vi "transform_axis_positions.vi"(6 "Current status":T1={"Axis names"=["X", "Y", "Z", "Rx", "Ry", "Rz"], "Axis positions"=[], "Pose"=[], "Timestamp"=0, "Ready"=FALSE, "Stopped"=FALSE} {"Pose" format="%#.4f"; "Axis positions" format="%#.4f"}, 8 "error in":errorcluster, 11 "Command":T2) -> (0 "error out":errorcluster, 1 "Absolute":bool, 2 "Axis positions":dbl[](array[numeric]), 3 "Axis enable":bool[](array[boolean]), 4 "Final status":T1={"Axis names"=["X", "Y", "Z", "Rx", "Ry", "Rz"], "Axis positions"=[], "Pose"=[], "Timestamp"=0, "Ready"=FALSE, "Stopped"=FALSE} {"Pose" format="%#.4f"; "Axis positions" format="%#.4f"})   [LabVIEW 2024]
uses:
  motion_command.ctl
  motion_status.ctl
  <vilib>/Analysis/baseanly.llb/Real A x B.vi
  <vilib>/Analysis/NI_AALBase.lvlib
panel:
  # "Do inverse kinematics, etc., to generate the inputs to the low-level motion drivers."
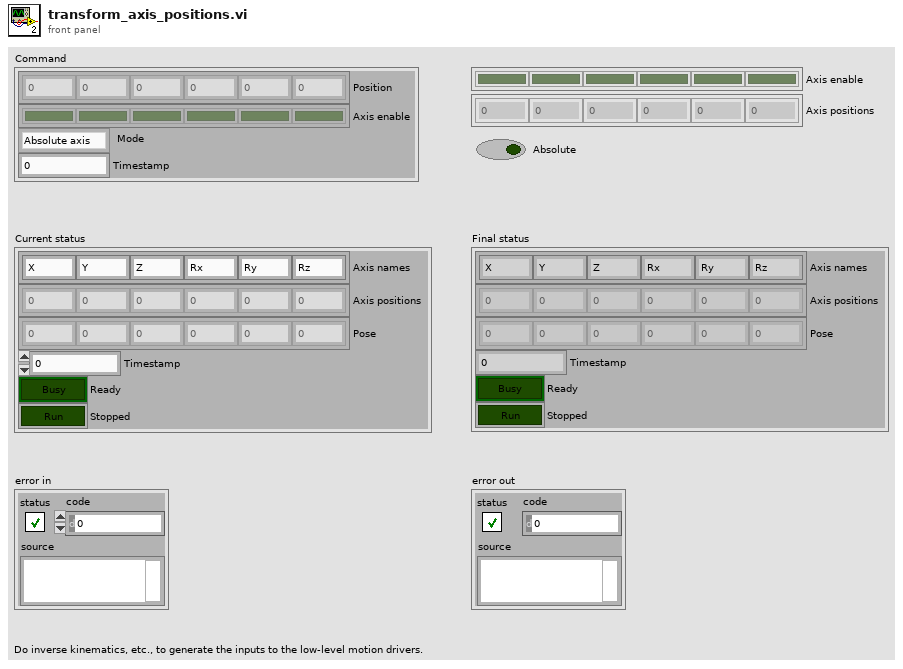
[diagram p1: front panel]
types:
  T1 = typedef "motion_status.ctl" = cluster{"Axis names":string[], "Axis positions":dbl[], "Pose":dbl[], "Timestamp":u32, "Ready":bool, "Stopped":bool}
  T2 = typedef "motion_command.ctl" = cluster{"Position":dbl[], "Axis enable":bool[], "Mode":enum16{"Absolute axis", "Relative axis", "Pose"}, "Timestamp":u32}
  T3 = typedef "NI_Matrix.lvlib/RealMatrix.ctl" = dbl[][]
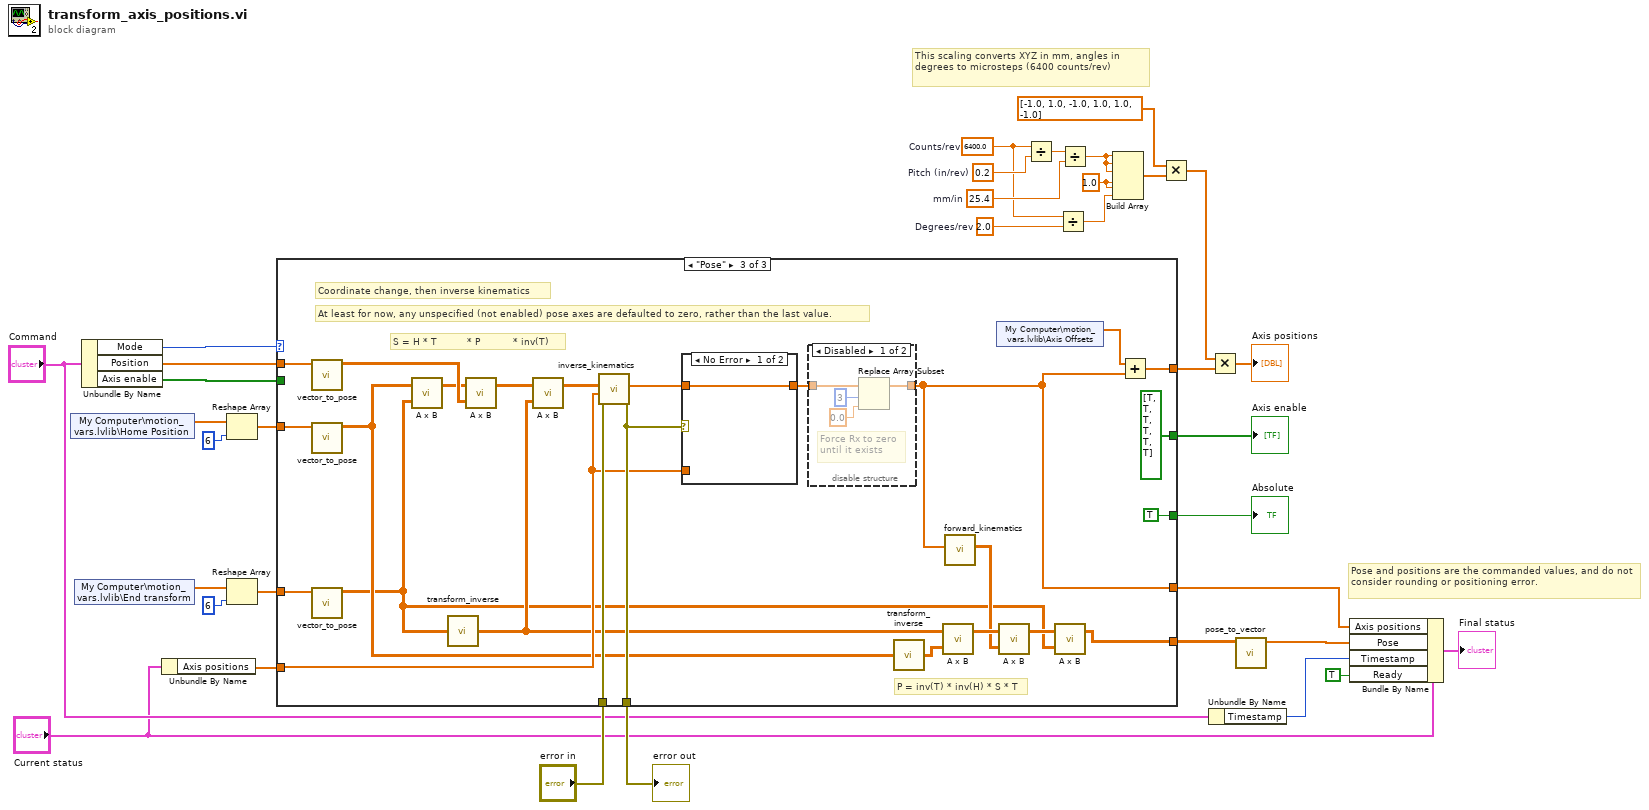
[diagram p0: block diagram]
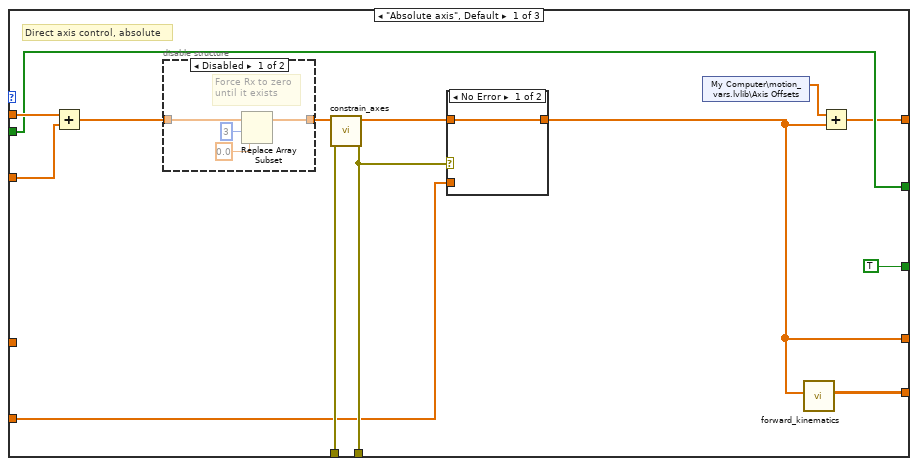
[diagram p2: hidden frame]
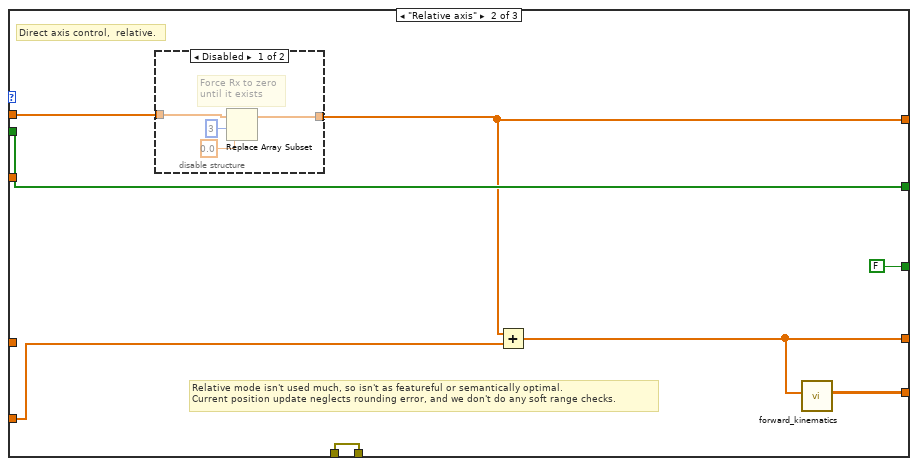
[diagram p5: hidden frame]
diagram:
  w12 = 1.0 ("element")
  w27 = 2.0  # Degrees/rev
  w33 = 25.4  # mm/in
  w34 = 0.2  # Pitch (in/rev)
  w28 = 6400.0  # Counts/rev
  # "Pose and positions are the commanded values, and do not consider rounding or positioning error."
  # "This scaling converts XYZ in mm, angles in degrees to microsteps (6400 counts/rev)"
  n1 = shared-variable "My Computer\\motion_vars.lvlib\\Home Position"() -> (w6:dbl[])  [unwired: 1 in, 1 out]
  n2 = shared-variable "My Computer\\motion_vars.lvlib\\End transform"() -> (w8:dbl[])  [unwired: 1 in, 1 out]
  n3 = Unbundle By Name("Command") -> ("Mode"=w25:enum16{"Absolute axis", "Relative axis", "Pose"}, "Position"=w24:dbl[], "Axis enable"=w23:bool[])
  n4 = Unbundle By Name("Current status") -> ("Axis positions"=w3:dbl[])
  n5 = Reshape Array(w6, 6 ("dimension size")) -> (w5:dbl[])
  n6 = Reshape Array(w8, 6 ("dimension size")) -> (w10:dbl[])
  n7 = case shown="\"Pose\"" w25 {
    tunnel: w24 -> [w49 w61 w94]
    tunnel: w10 -> [_ _ w93]
    tunnel: [w37 w60 w71] -> w1
    tunnel: w23 -> [w43 w64 _]
    tunnel: [w43 w64 bool[] [TRUE, TRUE, TRUE, TRUE, TRUE, TRUE] ("Axis enable")] -> w22
    tunnel: [TRUE FALSE TRUE] -> w21
    tunnel: w3 -> [w40 w59 w82]
    tunnel: [w42 w63 w85] -> w20
    tunnel: "error in" -> [w44 w63 w84]
    tunnel: [w45 w57 w74] -> w2
    tunnel: [w38 w58 w72] -> w16
    tunnel: w5 -> [w47 _ w83]
    frame "Absolute axis", Default {
      # "Direct axis control, absolute"
      n8 = Add(x=w49, y=w47) -> (x+y=w39:dbl[])
      n9 = disable-structure shown="Disabled" {
        disable-tunnel: [w51 w54] -> w46
        disable-tunnel: w39 -> [w50 w54]
        frame Disabled {
          # "Force Rx to zero\nuntil it exists"
          n10 = Replace Array Subset(array=w50, new element=0.0 ("new element/subarray"), index=3) -> (w51:dbl[])
        }
        frame Enabled {
        }
      }
      n11 = call "constrain_axes.vi"("error in"=w44, "Axis positions in"=w46) -> ("error out"=w42:errorcluster, "Axis positions out"=w41:dbl[])  [unwired: 7 in, 1 out]
      n12 = case shown="No Error" w42 {
        tunnel: [w55 w56] -> w38
        tunnel: w41 -> [w55 _]
        tunnel: w40 -> [_ w56]
        frame No Error {
        }
        frame Error {
        }
      }
      n13 = shared-variable "My Computer\\motion_vars.lvlib\\Axis Offsets"() -> (w36:dbl[])  [unwired: 1 in, 1 out]
      n14 = call "forward_kinematics.vi"("Axis positions"=w38) -> ("Pose"=w45:T3)  [unwired: 10 in]
      n15 = Add(x=w36, y=w38) -> (x+y=w37:dbl[])
    }
    frame "Relative axis" {
      # "Relative mode isn't used much, so isn't as featureful or semantically optimal.\nCurrent position update neglects rounding error, and we don't do any soft range checks."
      # "Direct axis control,  relative."
      n16 = disable-structure shown="Disabled" {
        disable-tunnel: w61 -> [w66 w69]
        disable-tunnel: [w65 w69] -> w60
        frame Disabled {
          # "Force Rx to zero\nuntil it exists"
          n17 = Replace Array Subset(array=w66, new element=0.0 ("new element/subarray"), index=3) -> (w65:dbl[])
        }
        frame Enabled {
        }
      }
      n18 = Add(x=w60, y=w59) -> (x+y=w58:dbl[])
      n19 = call "forward_kinematics.vi"("Axis positions"=w58) -> ("Pose"=w57:T3)  [unwired: 10 in]
    }
    frame "Pose" {
      # "P = inv(T) * inv(H) * S * T"
      # "S = H * T          * P           * inv(T)"
      # "At least for now, any unspecified (not enabled) pose axes are defaulted to zero, rather than the last value."
      # "Coordinate change, then inverse kinematics"
      n20 = call "vector_to_pose.vi"("Pose vector"=w94) -> ("Pose"=w89:T3)  [unwired: 10 in]
      n21 = call "vector_to_pose.vi"("Pose vector"=w83) -> ("Pose"=w79:T3)  [unwired: 10 in]
      n22 = call "vector_to_pose.vi"("Pose vector"=w93) -> ("Pose"=w75:T3)  [unwired: 10 in]
      n23 = call-poly <vilib>:"A x B.vi"("B"=w75, "A"=w79) -> ("A x B"=w88:T3)  [unwired: 1 out]
      n24 = call "transform_inverse.vi"("Transform"=w75) -> ("Inverse transform"=w81:T3)
      n25 = call-poly <vilib>:"A x B.vi"("B"=w89, "A"=w88) -> ("A x B"=w90:T3)  [unwired: 1 out]
      n26 = call-poly <vilib>:"A x B.vi"("B"=w81, "A"=w90) -> ("A x B"=w87:T3)  [unwired: 1 out]
      n27 = call "inverse_kinematics.vi"("error in"=w84, "Initial axis positions"=w82, "Pose"=w87) -> ("error out"=w85:errorcluster, "Axis positions"=w86:dbl[])  [unwired: 4 in, 3 out]
      n28 = case shown="No Error" w85 {
        tunnel: w86 -> [w100 _]
        tunnel: [w100 w101] -> w73
        tunnel: w82 -> [_ w101]
        frame No Error {
        }
        frame Error {
          # "No move if error"
        }
      }
      n29 = disable-structure shown="Disabled" {
        disable-tunnel: w73 -> [w96 w99]
        disable-tunnel: [w95 w99] -> w72
        frame Disabled {
          # "Force Rx to zero\nuntil it exists"
          n30 = Replace Array Subset(array=w96, new element=0.0 ("new element/subarray"), index=3) -> (w95:dbl[])
        }
        frame Enabled {
        }
      }
      n31 = call "transform_inverse.vi"("Transform"=w79) -> ("Inverse transform"=w80:T3)
      n32 = call-poly <vilib>:"A x B.vi"("B"=w80, "A"=w81) -> ("A x B"=w77:T3)  [unwired: 1 out]
      n33 = call "forward_kinematics.vi"("Axis positions"=w72) -> ("Pose"=w76:T3)  [unwired: 10 in]
      n34 = shared-variable "My Computer\\motion_vars.lvlib\\Axis Offsets"() -> (w70:dbl[])  [unwired: 1 in, 1 out]
      n35 = call-poly <vilib>:"A x B.vi"("B"=w76, "A"=w77) -> ("A x B"=w78:T3)  [unwired: 1 out]
      n36 = call-poly <vilib>:"A x B.vi"("B"=w75, "A"=w78) -> ("A x B"=w74:T3)  [unwired: 1 out]
      n37 = Add(x=w70, y=w72) -> (x+y=w71:dbl[])
    }
  }
  "Absolute" <- w21
  "Axis enable" <- w22
  "error out" <- w20
  n38 = Divide(x=w28, y=w34) -> (x/y=w32:dbl)
  n39 = Divide(x=w28, y=w27) -> (x/y=w11:dbl)
  n40 = Divide(x=w32, y=w33) -> (x/y=w30:dbl)
  n41 = Build Array(w30, w30, w30, w12, w12, w11) -> (w29:dbl[])
  n42 = Multiply(x=dbl[] [-1.0, 1.0, -1.0, 1.0, 1.0, -1.0] ("Axis positions"), y=w29) -> (x*y=w35:dbl[])
  n43 = Unbundle By Name("Command") -> ("Timestamp"=w14:u32)
  n44 = Multiply(x=w35, y=w1) -> (x*y=→"Axis positions":dbl[])
  n45 = call "pose_to_vector.vi"("Pose"=w2) -> ("Pose vector"=w17:dbl[])  [unwired: 10 in]
  n46 = Bundle By Name(cluster="Current status", "Axis positions"=w16, "Pose"=w17, "Timestamp"=w14, "Ready"=TRUE) -> (→"Final status":T1)
